vi "CreateVI.vi"(8 "error in (no error)":errorcluster, 9 "Dynamic Dispatch (T)":bool, 10 "Name":string, 11 "CreateInterface in":refnum<class "CreateInterface.lvclass">) -> (0 "error out":errorcluster, 3 "CreateInterface out":refnum<class "CreateInterface.lvclass">)   [LabVIEW 2020, in "Mermaid.lvlib" / "CreateInterface.lvclass"]
uses:
  CreateInterface.lvclass
  CreateInterface.lvclass/CreateInterface.ctl
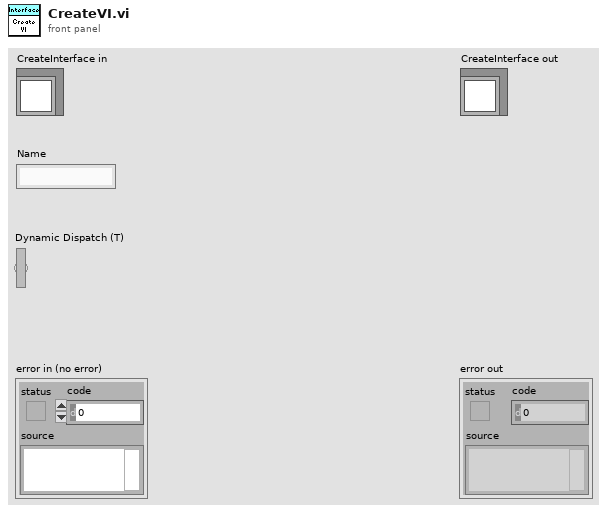
[diagram p1: front panel]
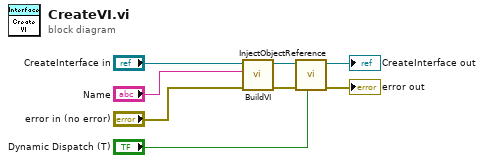
[diagram p0: block diagram]
diagram:
  n1 = call "BuildVI.vi"("error in (no error)"="error in (no error)", "Name"="Name", "CreateInterface in"="CreateInterface in") -> ("error out"=w4:errorcluster, "CreateInterface out"=w5:refnum<class "CreateInterface.lvclass">)  [unwired: 7 in]
  n2 = call "InjectObjectReference.vi"("Dynamic Dispatch"="Dynamic Dispatch (T)", "error in (no error)"=w4, "CreateInterface in"=w5) -> ("error out"=→"error out":errorcluster, "CreateInterface out"=→"CreateInterface out":refnum<class "CreateInterface.lvclass">)  [unwired: 7 in]
